vi "Логи_АЦП.vi"() -> ()   [LabVIEW 2013]
panel:
  in  "Tab Control":T1(tab)
  out "XY Graph 2":cluster{dbl[], dbl[]}[](graph)
  out "XY Graph 3":cluster{dbl[], dbl[]}[](graph)
  out "?":cluster{dbl[], dbl[]}[](graph)
  out "ID параметров":u8[](array[numeric])
  out "Длина заголовка":i32
  out "Заголовок":string
  out "Количество параметров":u8
  out "size (in bytes)":i64
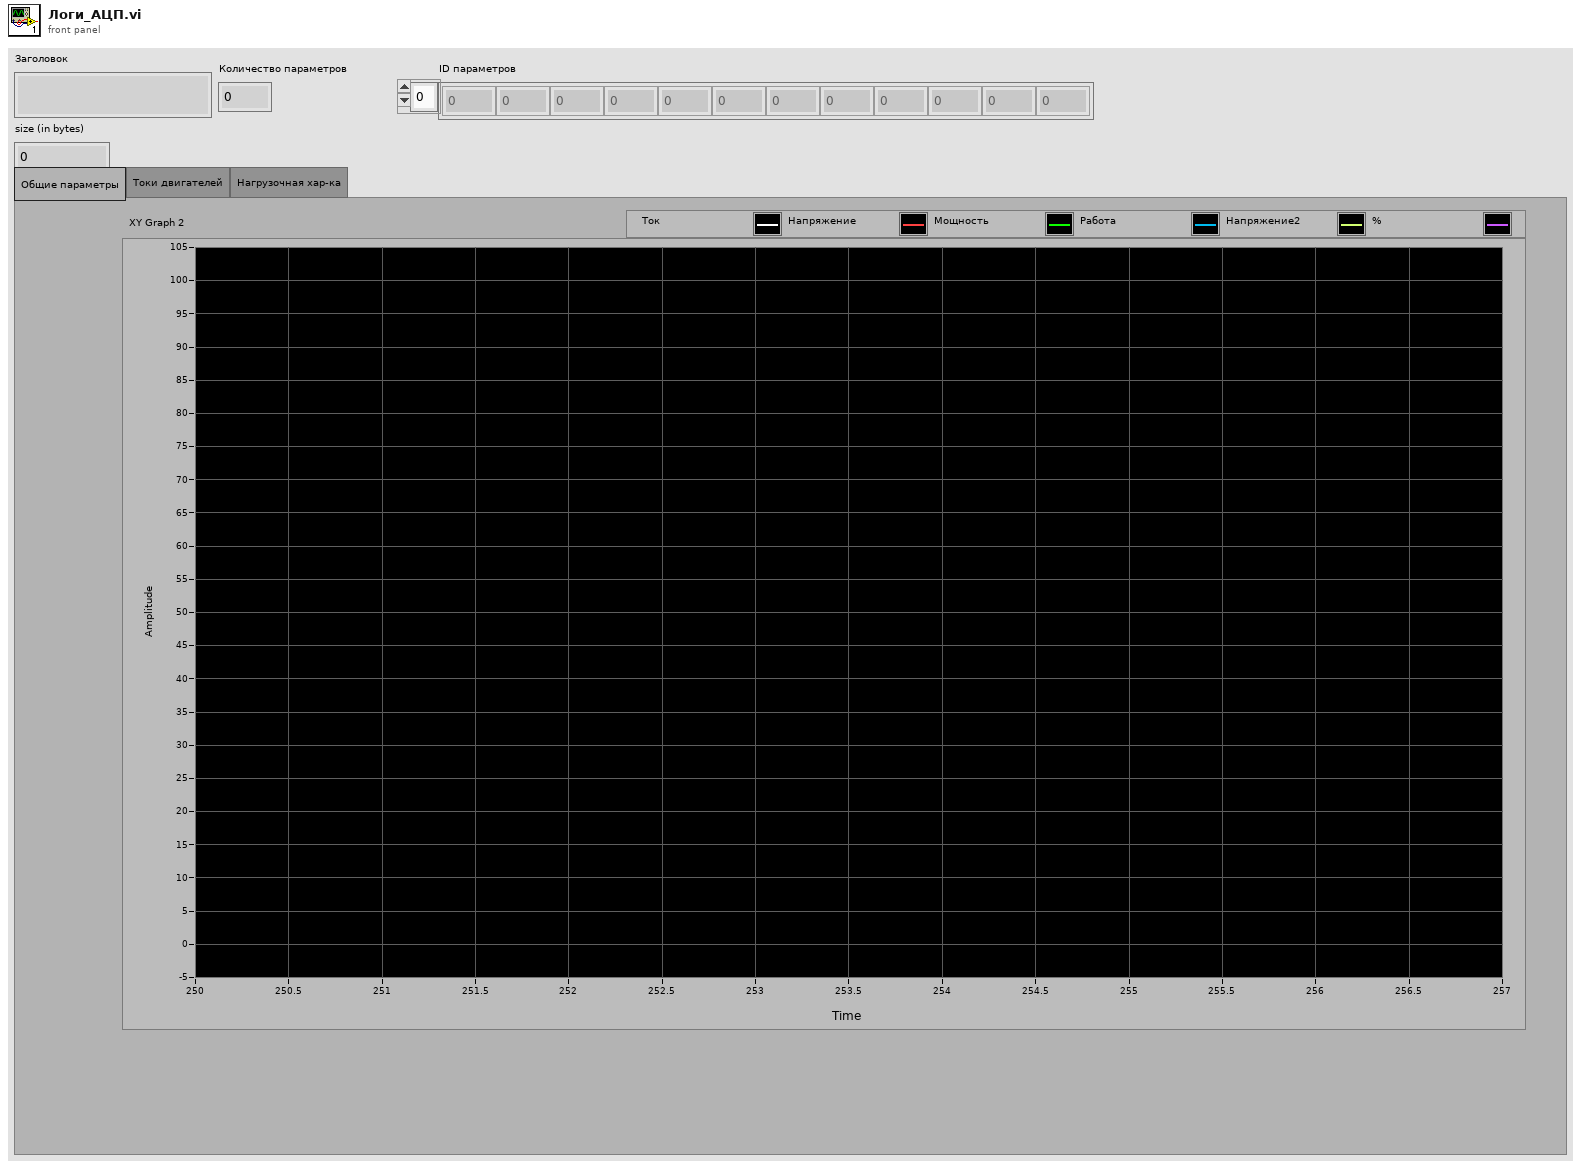
[diagram p1: front panel]
types:
  T1 = enum32{"Общие параметры", "Токи двигателей", "Нагрузочная хар-ка"}
  T2 = enum16{"open", "replace", "create", "open or create", "replace or create", "replace or create with confirmation"}
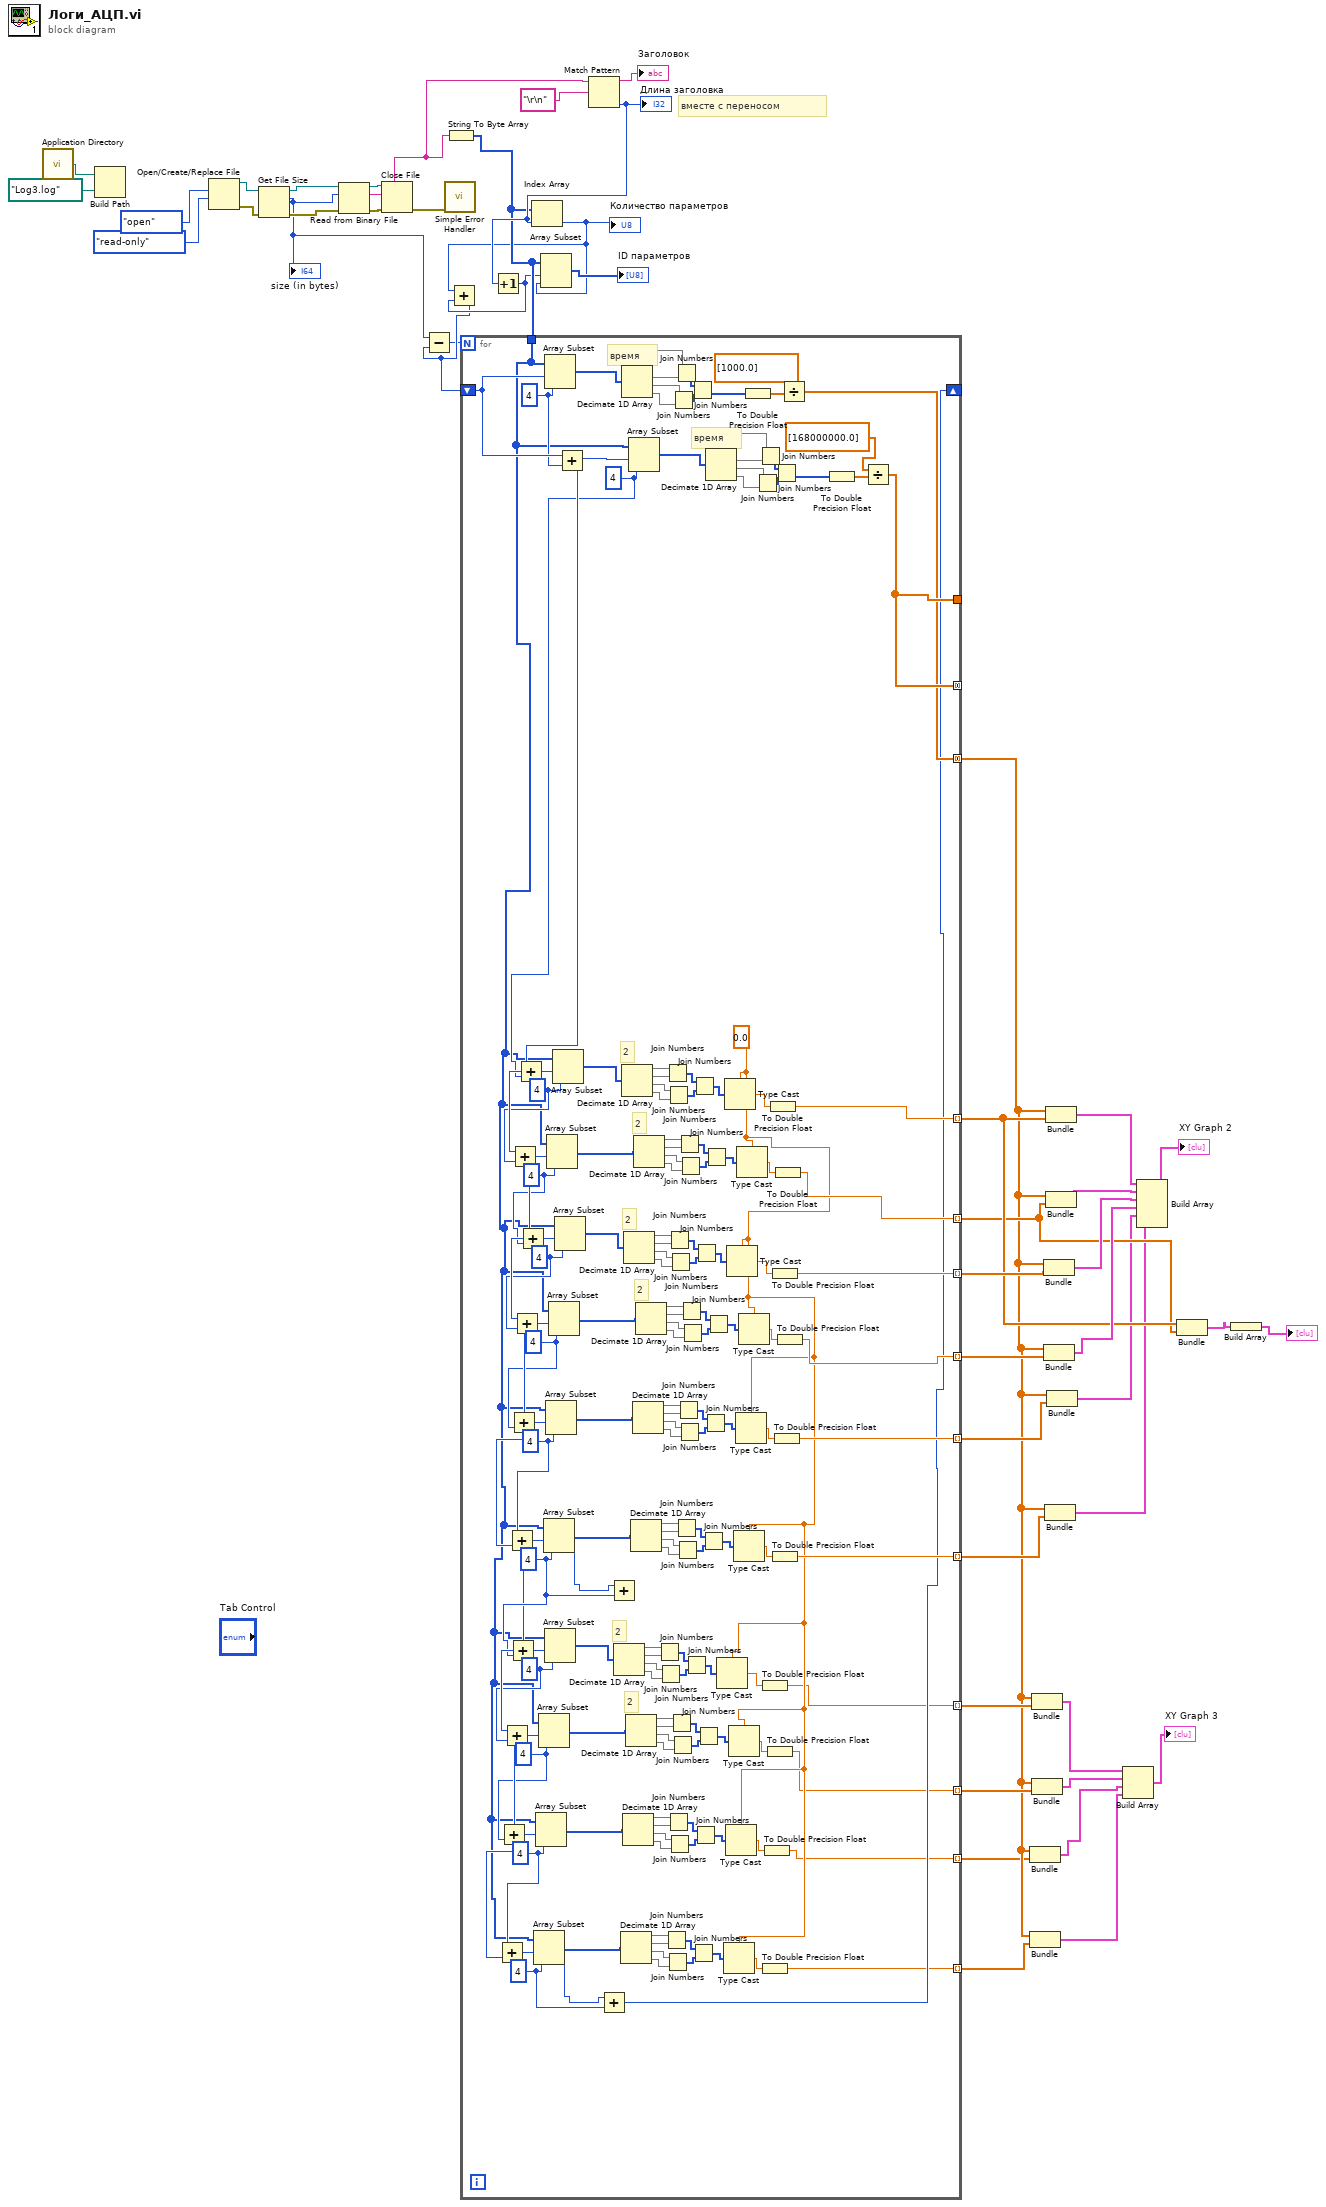
[diagram p0: block diagram]
diagram:
  # "вместе с переносом"
  n1 = call <vilib>:"Application Directory.vi"() -> ("Application Directory"=w44:path)
  n2 = Build Path(base path=w44, name or relative path=path "Log3.log" ("default name")) -> ()  [unwired: 1 out]
  n3 = Open/Create/Replace File(operation (0:open)=T2."open", access (0:read/write)=enum16{"read/write", "read-only", "write-only"}."read-only") -> (refnum out=w41:refnum<file>, error out=w39:errorcluster)  [unwired: 4 in, 1 out]
  n4 = Get File Size(file=w41, error in=w39) -> (refnum out=w40:refnum<file>, size (in bytes)=w31:i64, 0:w38:errorcluster)
  "size (in bytes)" <- w31
  n5 = Read from Binary File(8:w38, 10:w31, 11:w40) -> (0:w42:errorcluster, 2:w37:string, 3:w43:refnum<file>)  [unwired: 3 in, 1 out]
  n6 = Close File(refnum=w43, error in=w42) -> (error out=w47:errorcluster)  [unwired: 1 out]
  n7 = call <vilib>:"Simple Error Handler.vi"("error in (no error)"=w47) -> ()  [unwired: 4 in, 5 out]
  n8 = String To Byte Array(string=w37) -> (unsigned byte array=w32:u8[])
  n9 = Match Pattern(string=w37, regular expression="\r\n" ("format string")) -> (before substring=→"Заголовок":string, offset past match=w34:i32)  [unwired: 1 in, 2 out]
  "Длина заголовка" <- w34
  n10 = Increment(x=w34) -> (x+1=w29:i32)
  n11 = Index Array(array=w32, index=w34) -> (element=w30:u8)
  "Количество параметров" <- w30
  n12 = Add(x=w30, y=w29) -> (x+y=w28:i32)
  n13 = Subtract(x=w31, y=w28) -> (x-y=w27:i64)
  n14 = for {
    N: w27 -> [_]
    tunnel: w32 -> [w53]
    shift-right: [w56] -> _
    shift-left: w28 -> [w178]
    tunnel: [w174] -> _ mode=concatenating
    tunnel: [w174] -> _
    tunnel: [w153] -> w16 mode=indexing
    tunnel: [w152] -> w15 mode=indexing
    tunnel: [w129] -> w22 mode=indexing
    tunnel: [w128] -> w21 mode=indexing
    tunnel: [w116] -> w14 mode=indexing
    tunnel: [w113] -> w8 mode=concatenating
    tunnel: [w101] -> w12 mode=indexing
    tunnel: [w51] -> w10 mode=indexing
    tunnel: [w50] -> w9 mode=indexing
    tunnel: [w49] -> w7 mode=indexing
    tunnel: [w48] -> w6 mode=indexing
    w59 = 4 ("length")
    w58 = 4 ("length")
    w70 = 4 ("length")
    w99 = 4 ("length")
    w55 = 4 ("length")
    w103 = 4 ("length")
    w117 = 4 ("length")
    w150 = 4 ("length")
    w52 = sgl 0.0
    w130 = 4 ("length")
    w172 = 4 ("length")
    w114 = 4 ("length")
    w177 = 4 ("length")
    # "2"
    # "2"
    # "2"
    # "2"
    # "2"
    # "2"
    # "время"
    # "время"
    n15 = Array Subset(array=w53, index=w178, length=w177) -> (w190:u8[])
    n16 = Add(x=w178, y=w177) -> (x+y=w115:i32)
    n17 = Add(x=w115, y=w114) -> (x+y=w173:i32)
    n18 = Add(x=w173, y=w172) -> (x+y=w131:i32)
    n19 = Add(x=w131, y=w130) -> (x+y=w151:i32)
    n20 = Add(x=w151, y=w150) -> (x+y=w118:i32)
    n21 = Add(x=w118, y=w117) -> (x+y=w102:i32)
    n22 = Add(x=w103, y=w102) -> (x+y=w54:i32)
    n23 = Add(x=w54, y=w55) -> (x+y=w100:i32)
    n24 = Add(x=w100, y=w99) -> (x+y=w71:i32)
    n25 = Add(x=w71, y=w70) -> (x+y=w57:i32)
    n26 = Add(x=w58, y=w57) -> (x+y=w60:i32)
    n27 = Array Subset(array=w53, index=w60, length=w59) -> (w63:u8[])
    n28 = Array Subset(array=w53, index=w57, length=w58) -> (w74:u8[])
    n29 = Array Subset(array=w53, index=w71, length=w70) -> (w85:u8[])
    n30 = Array Subset(array=w53, index=w54, length=w55) -> (w106:u8[])
    n31 = Array Subset(array=w53, index=w100, length=w99) -> (w96:u8[])
    n32 = Array Subset(array=w53, index=w102, length=w103) -> (w121:u8[])
    n33 = Array Subset(array=w53, index=w131, length=w130) -> (w158:u8[])
    n34 = Array Subset(array=w53, index=w118, length=w117) -> (w136:u8[])
    n35 = Array Subset(array=w53, index=w173, length=w172) -> (w169:u8[])
    n36 = Array Subset(array=w53, index=w151, length=w150) -> (w147:u8[])
    n37 = Add(x=w60, y=w59) -> (x+y=w56:i32)
    n38 = Add(x=w54, y=w55) -> ()  [unwired: 1 out]
    n39 = Decimate 1D Array(w96) -> (w97:u8[], w98:u8[], w95:u8[], w94:u8[])
    n40 = Decimate 1D Array(w63) -> (w68:u8[], w69:u8[], w67:u8[], w66:u8[])
    n41 = Decimate 1D Array(w190) -> (w192:u8[], w193:u8[], w194:u8[], w195:u8[])
    n42 = Decimate 1D Array(w169) -> (w170:u8[], w171:u8[], w168:u8[], w167:u8[])
    n43 = Decimate 1D Array(w74) -> (w79:u8[], w80:u8[], w78:u8[], w77:u8[])
    n44 = Decimate 1D Array(w147) -> (w148:u8[], w149:u8[], w146:u8[], w145:u8[])
    n45 = Decimate 1D Array(w85) -> (w90:u8[], w91:u8[], w89:u8[], w88:u8[])
    n46 = Array Subset(array=w53, index=w115, length=w114) -> (w180:u8[])
    n47 = Decimate 1D Array(w106) -> (w111:u8[], w112:u8[], w110:u8[], w109:u8[])
    n48 = Decimate 1D Array(w121) -> (w126:u8[], w127:u8[], w125:u8[], w124:u8[])
    n49 = Decimate 1D Array(w158) -> (w163:u8[], w164:u8[], w162:u8[], w161:u8[])
    n50 = Decimate 1D Array(w136) -> (w141:u8[], w142:u8[], w140:u8[], w139:u8[])
    n51 = Join Numbers(hi=w97, lo=w98) -> ((hi.lo)=w93:u16[])
    n52 = Join Numbers(hi=w95, lo=w94) -> ((hi.lo)=w92:u16[])
    n53 = Join Numbers(hi=w68, lo=w69) -> ((hi.lo)=w65:u16[])
    n54 = Join Numbers(hi=w170, lo=w171) -> ((hi.lo)=w166:u16[])
    n55 = Join Numbers(hi=w67, lo=w66) -> ((hi.lo)=w64:u16[])
    n56 = Join Numbers(hi=w168, lo=w167) -> ((hi.lo)=w165:u16[])
    n57 = Join Numbers(hi=w79, lo=w80) -> ((hi.lo)=w76:u16[])
    n58 = Join Numbers(hi=w148, lo=w149) -> ((hi.lo)=w144:u16[])
    n59 = Join Numbers(hi=w78, lo=w77) -> ((hi.lo)=w75:u16[])
    n60 = Join Numbers(hi=w146, lo=w145) -> ((hi.lo)=w143:u16[])
    n61 = Join Numbers(hi=w90, lo=w91) -> ((hi.lo)=w87:u16[])
    n62 = Join Numbers(hi=w89, lo=w88) -> ((hi.lo)=w86:u16[])
    n63 = Join Numbers(hi=w194, lo=w195) -> ((hi.lo)=w191:u16[])
    n64 = Join Numbers(hi=w192, lo=w193) -> ((hi.lo)=w196:u16[])
    n65 = Join Numbers(hi=w111, lo=w112) -> ((hi.lo)=w108:u16[])
    n66 = Join Numbers(hi=w110, lo=w109) -> ((hi.lo)=w107:u16[])
    n67 = Join Numbers(hi=w126, lo=w127) -> ((hi.lo)=w123:u16[])
    n68 = Join Numbers(hi=w163, lo=w164) -> ((hi.lo)=w160:u16[])
    n69 = Join Numbers(hi=w125, lo=w124) -> ((hi.lo)=w122:u16[])
    n70 = Join Numbers(hi=w162, lo=w161) -> ((hi.lo)=w159:u16[])
    n71 = Join Numbers(hi=w141, lo=w142) -> ((hi.lo)=w138:u16[])
    n72 = Join Numbers(hi=w140, lo=w139) -> ((hi.lo)=w137:u16[])
    n73 = Join Numbers(hi=w93, lo=w92) -> ((hi.lo)=w82:u32[])
    n74 = Join Numbers(hi=w196, lo=w191) -> ((hi.lo)=w187:u32[])
    n75 = Join Numbers(hi=w65, lo=w64) -> ((hi.lo)=w62:u32[])
    n76 = Join Numbers(hi=w166, lo=w165) -> ((hi.lo)=w155:u32[])
    n77 = Join Numbers(hi=w76, lo=w75) -> ((hi.lo)=w73:u32[])
    n78 = Join Numbers(hi=w144, lo=w143) -> ((hi.lo)=w133:u32[])
    n79 = Join Numbers(hi=w87, lo=w86) -> ((hi.lo)=w84:u32[])
    n80 = Join Numbers(hi=w108, lo=w107) -> ((hi.lo)=w105:u32[])
    n81 = Join Numbers(hi=w123, lo=w122) -> ((hi.lo)=w120:u32[])
    n82 = Join Numbers(hi=w160, lo=w159) -> ((hi.lo)=w157:u32[])
    n83 = Join Numbers(hi=w138, lo=w137) -> ((hi.lo)=w135:u32[])
    n84 = Decimate 1D Array(w180) -> (w182:u8[], w183:u8[], w184:u8[], w185:u8[])
    n85 = Type Cast(type=w52, x=w82) -> (*(type *) &x=w81:sgl)
    n86 = Type Cast(type=w52, x=w62) -> (*(type *) &x=w61:sgl)
    n87 = Type Cast(type=w52, x=w155) -> (*(type *) &x=w154:sgl)
    n88 = Type Cast(type=w52, x=w73) -> (*(type *) &x=w72:sgl)
    n89 = Type Cast(type=w52, x=w133) -> (*(type *) &x=w132:sgl)
    n90 = Type Cast(type=w52, x=w84) -> (*(type *) &x=w83:sgl)
    n91 = Type Cast(type=w52, x=w105) -> (*(type *) &x=w104:sgl)
    n92 = Type Cast(type=w52, x=w120) -> (*(type *) &x=w119:sgl)
    n93 = Type Cast(type=w52, x=w157) -> (*(type *) &x=w156:sgl)
    n94 = Type Cast(type=w52, x=w135) -> (*(type *) &x=w134:sgl)
    n95 = To Double Precision Float(number=w187) -> (double precision float=w189:dbl[])
    n96 = Join Numbers(hi=w184, lo=w185) -> ((hi.lo)=w181:u16[])
    n97 = Join Numbers(hi=w182, lo=w183) -> ((hi.lo)=w186:u16[])
    n98 = To Double Precision Float(number=w81) -> (double precision float=w51:dbl)
    n99 = To Double Precision Float(number=w61) -> (double precision float=w48:dbl)
    n100 = To Double Precision Float(number=w72) -> (double precision float=w49:dbl)
    n101 = To Double Precision Float(number=w83) -> (double precision float=w50:dbl)
    n102 = To Double Precision Float(number=w154) -> (double precision float=w153:dbl)
    n103 = To Double Precision Float(number=w132) -> (double precision float=w129:dbl)
    n104 = To Double Precision Float(number=w104) -> (double precision float=w101:dbl)
    n105 = Join Numbers(hi=w186, lo=w181) -> ((hi.lo)=w179:u32[])
    n106 = To Double Precision Float(number=w119) -> (double precision float=w116:dbl)
    n107 = To Double Precision Float(number=w156) -> (double precision float=w152:dbl)
    n108 = To Double Precision Float(number=w134) -> (double precision float=w128:dbl)
    n109 = Divide(x=w189, y=dbl[] [1000.0]) -> (x/y=w113:dbl[])
    n110 = To Double Precision Float(number=w179) -> (double precision float=w176:dbl[])
    n111 = Divide(x=dbl[] [168000000.0] ("y"), y=w176) -> (x/y=w174:dbl[])
  }
  n112 = Array Subset(array=w32, index=w29, length=w30) -> (→"ID параметров":u8[])
  n113 = Bundle(w8, w7) -> (w3:cluster{dbl[], dbl[]})  [unwired: 1 in]
  n114 = Bundle(w8, w6) -> (w2:cluster{dbl[], dbl[]})  [unwired: 1 in]
  n115 = Bundle(w8, w10) -> (w5:cluster{dbl[], dbl[]})  [unwired: 1 in]
  n116 = Bundle(w8, w9) -> (w4:cluster{dbl[], dbl[]})  [unwired: 1 in]
  n117 = Bundle(w8, w22) -> (w20:cluster{dbl[], dbl[]})  [unwired: 1 in]
  n118 = Bundle(w8, w21) -> (w19:cluster{dbl[], dbl[]})  [unwired: 1 in]
  n119 = Bundle(w8, w12) -> (w11:cluster{dbl[], dbl[]})  [unwired: 1 in]
  n120 = Bundle(w8, w16) -> (w25:cluster{dbl[], dbl[]})  [unwired: 1 in]
  n121 = Bundle(w8, w15) -> (w24:cluster{dbl[], dbl[]})  [unwired: 1 in]
  n122 = Bundle(w8, w14) -> (w13:cluster{dbl[], dbl[]})  [unwired: 1 in]
  n123 = Build Array(w5, w4, w3, w2) -> (→"XY Graph 3":cluster{dbl[], dbl[]}[])
  n124 = Build Array(w25, w24, w20, w19, w13, w11) -> (→"XY Graph 2":cluster{dbl[], dbl[]}[])
  n125 = Bundle(w16, w15) -> (w17:cluster{dbl[], dbl[]})  [unwired: 1 in]
  n126 = Build Array(w17) -> (→"?":cluster{dbl[], dbl[]}[])
